vi "sub_reconnect_attempt.vi"(4 "timeout for GET routes":i32=1000, 6 "daq.io API Base":string, 7 "Account ID":string, 8 "error in (no error)":errorcluster, 9 "Device Key":string, 10 "Credentials":T1, 11 "daq.io type in OLD":T2={"daq.io ref"=refnum, "daq.io API Base"="", "Device Key"="", "Account ID"="", "online"=TRUE, "SSL"=FALSE}) -> (0 "error out":errorcluster, 2 "logged in?":bool, 3 "daq.io type out":T2={"daq.io ref"=refnum, "daq.io API Base"="", "Device Key"="", "Account ID"="", "online"=TRUE, "SSL"=FALSE})   [LabVIEW 2013, in "daqio minimal.lvlib"]
uses:
  daqio minimal.lvlib
  _typedefs/daqio-Type.ctl
  <vilib>/httpClient/ClientHandle.ctl
  _typedefs/daqio-Credentials.ctl
  _typedefs/connection_FGV_commands.ctl
  <vilib>/httpClient/LabVIEWHTTPClient.lvlib
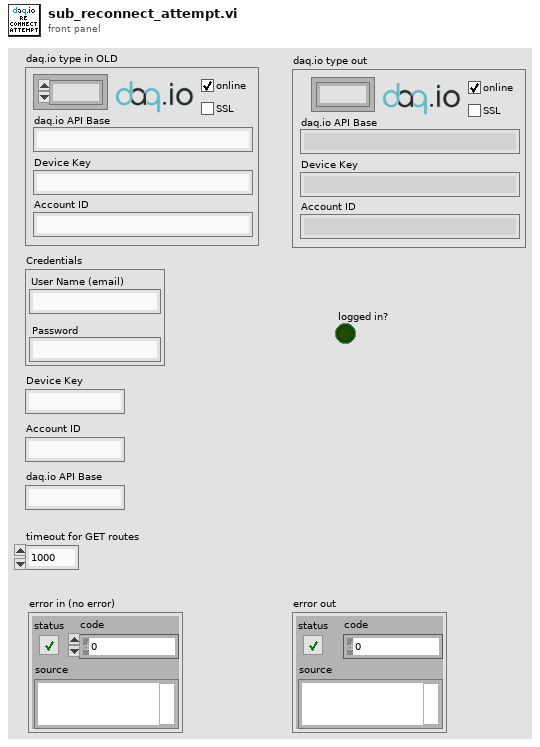
[diagram p1: front panel]
types:
  T1 = typedef "daqio minimal.lvlib/daqio-Credentials.ctl" = cluster{"User Name (email)":string, "Password":string}
  T2 = typedef "daqio minimal.lvlib/daqio-Type.ctl" = cluster{"daq.io ref":T3, "daq.io API Base":string, "Device Key":string, "Account ID":string, "online":bool, "SSL":bool}
  T3 = typedef "LabVIEWHTTPClient.lvlib/ClientHandle.ctl" = refnum<k1>
  T4 = typedef "daqio minimal.lvlib/connection_FGV_commands.ctl" = enum16{"Set Conn Stat", "Save Type", "Get Type from File", "Set Type", "Set Buffer", "Get"}
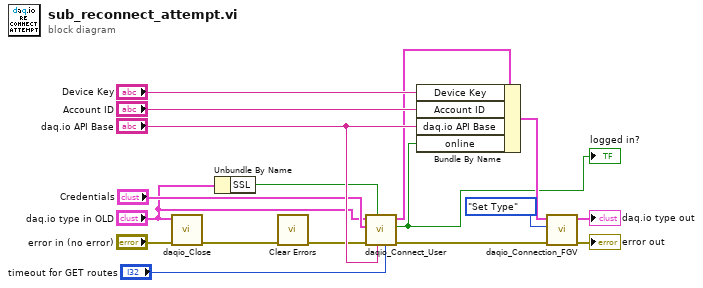
[diagram p0: block diagram]
diagram:
  n1 = call "daqio_Close.vi"("error in (no error)"="error in (no error)", "daq.io type"="daq.io type in OLD") -> ("error out"=w15:errorcluster)  [unwired: 9 in]
  n2 = Unbundle By Name("daq.io type in OLD") -> ("SSL"=w3:bool)
  n3 = call <vilib>:"Clear Errors.vi"("error in (no error)"=w15) -> ("error out"=w5:errorcluster)  [unwired: 6 in]
  n4 = call "daqio_Connect_User.vi"("timeout for GET routes"="timeout for GET routes", "daq.io API base"="daq.io API Base", "Use SSL"=w3, "error in (no error)"=w5, "Credentials"="Credentials", "daq.io type in"="daq.io type in OLD") -> ("error out"=w6:errorcluster, "logged in?"=w4:bool, "daq.io type"=w7:T2)  [unwired: 3 in]
  "logged in?" <- w4
  n5 = Bundle By Name(cluster=w7, "Device Key"="Device Key", "Account ID"="Account ID", "daq.io API Base"="daq.io API Base", "online"=w4) -> (w12:T2)
  n6 = call "daqio_Connection_FGV.vi"("error in"=w6, "Enum"=connection_FGV_commands."Set Type", "daq.io type in"=w12) -> ("error out"=→"error out":errorcluster, "daq.io type out"=→"daq.io type out":T2)  [unwired: 5 in, 2 out]
